vi "RunDuringExperiment.vi"() -> ()   [LabVIEW 2012]
uses:
  GlobalVars.vi
panel:
  in  "Average N Reference Frames":dbl=1.0 min=1.0
  in  "Position Shift Limit (Microns)":dbl=3.0 min=0.0
  out "Out of Limits":bool
  in  "Display Trace Offset (Microns)":dbl=5.0 min=0.0
  out "Z2":dbl[][](graph)=[[-0.26565398159854325, 5.190448689568315]]
  out "Y2":dbl[][](graph)=[[-0.26565398159854325, 5.190448689568315]]
  out "X2":dbl[][](graph)=[[-0.26565398159854325, 5.190448689568315]]
  out "Z1":dbl[][](graph)=[[0.023788275848097486, 4.878801842612402]]
  out "Y1":dbl[][](graph)=[[0.023788275848097486, 4.878801842612402]]
  out "X1":dbl[][](graph)=[[0.023788275848097486, 4.878801842612402]]
  # "X-Y Orthogonal Plane"
  # "X-Y Plane"
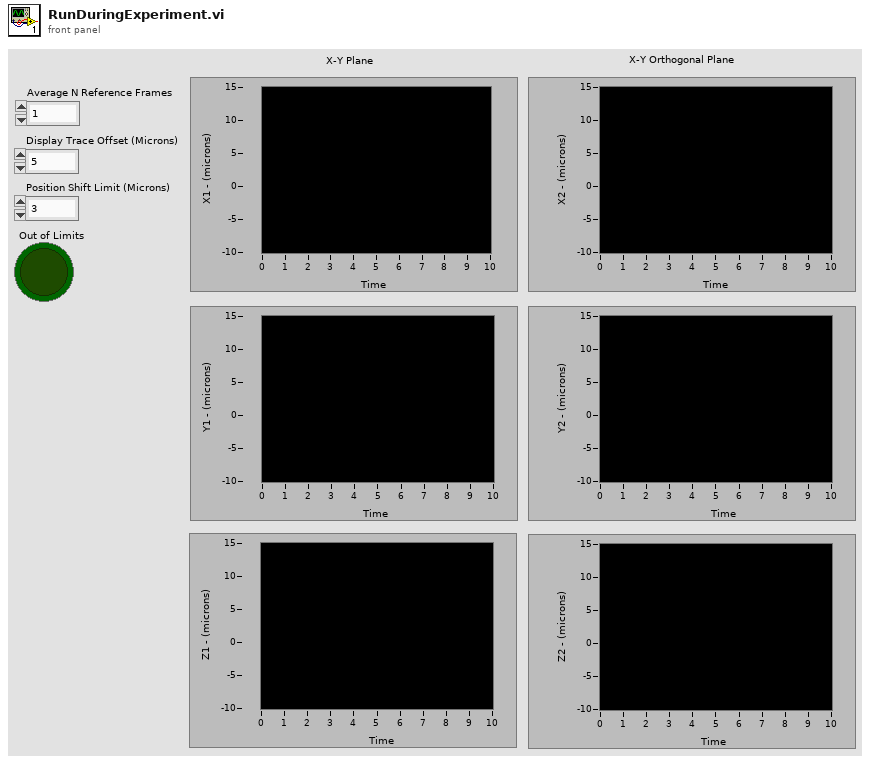
[diagram p1: front panel]
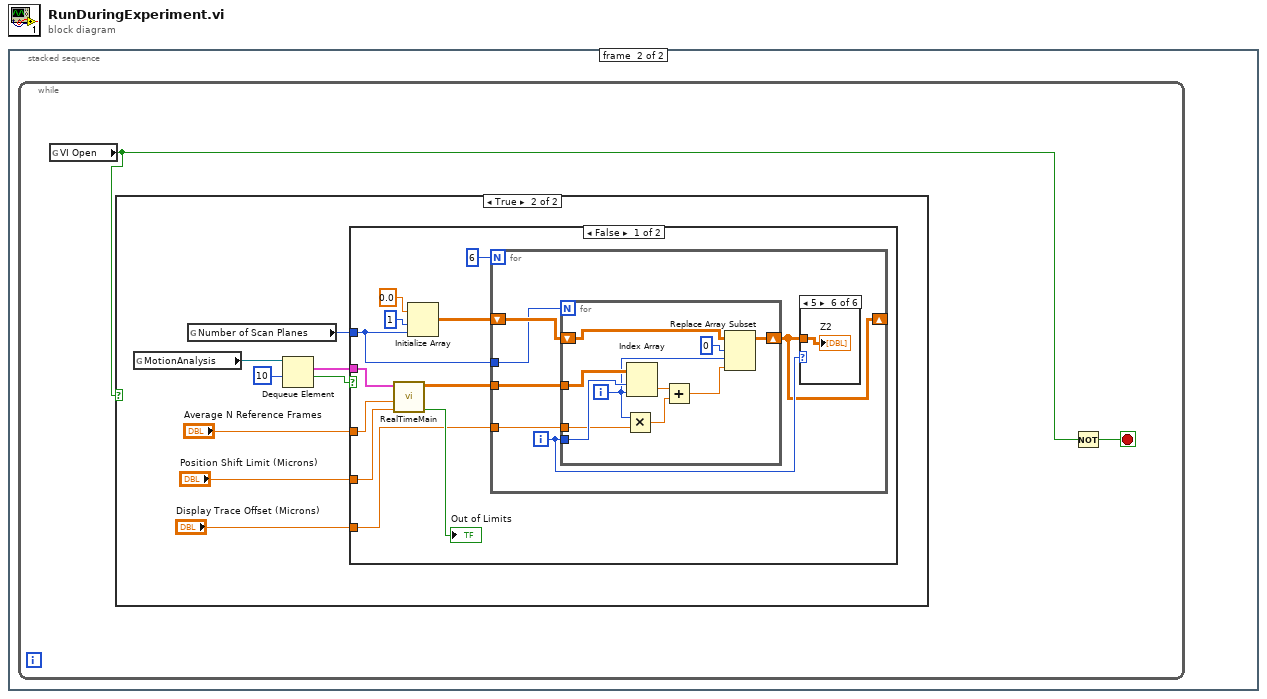
[diagram p0: block diagram]
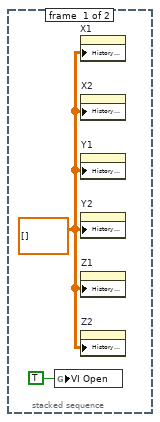
[diagram p2: hidden frame]
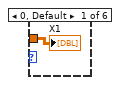
[diagram p4: hidden frame]
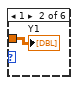
[diagram p5: hidden frame]
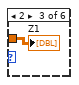
[diagram p6: hidden frame]
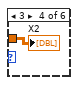
[diagram p7: hidden frame]
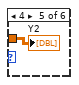
[diagram p8: hidden frame]
diagram:
  n1 = stacked-sequence {
    frame #0 {
      w1 = dbl[][] [] ("History Data")
      n2 = global write "GlobalVars.vi" "VI Open"(TRUE ("VI Open")) -> ()
      n3 = property on="X1" class="WFChart (strict)"("History Data"=w1) -> ()  [unwired: 2 in, 2 out]
      n4 = property on="X2" class="WFChart (strict)"("History Data"=w1) -> ()  [unwired: 2 in, 2 out]
      n5 = property on="Y1" class="WFChart (strict)"("History Data"=w1) -> ()  [unwired: 2 in, 2 out]
      n6 = property on="Y2" class="WFChart (strict)"("History Data"=w1) -> ()  [unwired: 2 in, 2 out]
      n7 = property on="Z1" class="WFChart (strict)"("History Data"=w1) -> ()  [unwired: 2 in, 2 out]
      n8 = property on="Z2" class="WFChart (strict)"("History Data"=w1) -> ()  [unwired: 2 in, 2 out]
    }
    frame #1 {
      n9 = while {
        stop <- w4 stop-if-true
        n10 = global read "GlobalVars.vi" "VI Open"() -> (w3:bool)
        n11 = case shown="True" w3 {
          frame False {
          }
          frame True {
            n12 = global read "GlobalVars.vi" "MotionAnalysis"() -> (w9:refnum<queue>)
            n13 = global read "GlobalVars.vi" "Number of Scan Planes"() -> (w7:i32)
            n14 = Dequeue Element(queue=w9, timeout in ms (-1)=10) -> (element=w8:cluster{dbl[][], dbl, dbl, dbl, dbl, dbl, dbl}[], timed out?=w6:bool)  [unwired: 1 in, 2 out]
            n15 = case shown="False" w6 {
              tunnel: "Position Shift Limit (Microns)" -> [w18 _]
              tunnel: "Display Trace Offset (Microns)" -> [w17 _]
              tunnel: "Average N Reference Frames" -> [w15 _]
              tunnel: w8 -> [w14 _]
              tunnel: w7 -> [w13 _]
              frame False {
                n16 = call "RealTimeMain.vi"("Threshold (microns)"=w18, "For Reference (frames)"=w15, "Motion Data"=w14) -> ("Stop Recording"=→"Out of Limits":bool, "Array"=w20:dbl[][])  [unwired: 7 in]
                n17 = Initialize Array(0.0 ("element"), 1 ("dimension size"), w13) -> (w21:dbl[][])
                n18 = for {
                  N: 6 -> [_]
                  tunnel: w20 -> [w28]
                  tunnel: w17 -> [w25]
                  tunnel: w13 -> [w24]
                  shift-right: [w26] -> _
                  shift-left: w21 -> [w29]
                  i -> [w27]
                  n19 = for {
                    N: w24 -> [_]
                    tunnel: w28 -> [w39]
                    tunnel: w27 -> [w38]
                    tunnel: w25 -> [w33]
                    shift-right: [w35] -> w26
                    shift-left: w29 -> [w37]
                    i -> [w34]
                    n20 = Multiply(x=w34, y=w33) -> (x*y=w32:dbl)
                    n21 = Index Array(array=w39, index (row)=w38, index (col)=w34) -> (element=w31:dbl)
                    n22 = Add(x=w31, y=w32) -> (x+y=w30:dbl)
                    n23 = Replace Array Subset(array=w37, new element=w30, index (row)=0, index (col)=w34) -> (w35:dbl[][])
                  }
                  n24 = case shown="5" w27 {
                    tunnel: w26 -> [w40 w41 w42 w43 w44 w45]
                    frame 0, Default {
                      "X1" <- w40
                    }
                    frame 1 {
                      "Y1" <- w41
                    }
                    frame 2 {
                      "Z1" <- w42
                    }
                    frame 3 {
                      "X2" <- w43
                    }
                    frame 4 {
                      "Y2" <- w44
                    }
                    frame 5 {
                      "Z2" <- w45
                    }
                  }
                }
              }
              frame True {
              }
            }
          }
        }
        n25 = Not(x=w3) -> (.not. x?=w4:bool)
      }
    }
  }
